vi "SafeMove.vi"(0 "Total Distance (mm)":dbl, 5 "Forward/Reverse":bool, 7 "Calibration Constant":dbl, 9 "Axis#":i16 min=0 max=2 step=1) -> (11 "5V Indicator":bool)   [LabVIEW 2017]
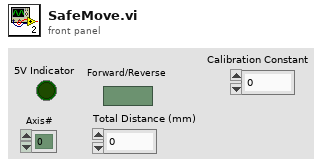
[diagram p1: front panel]
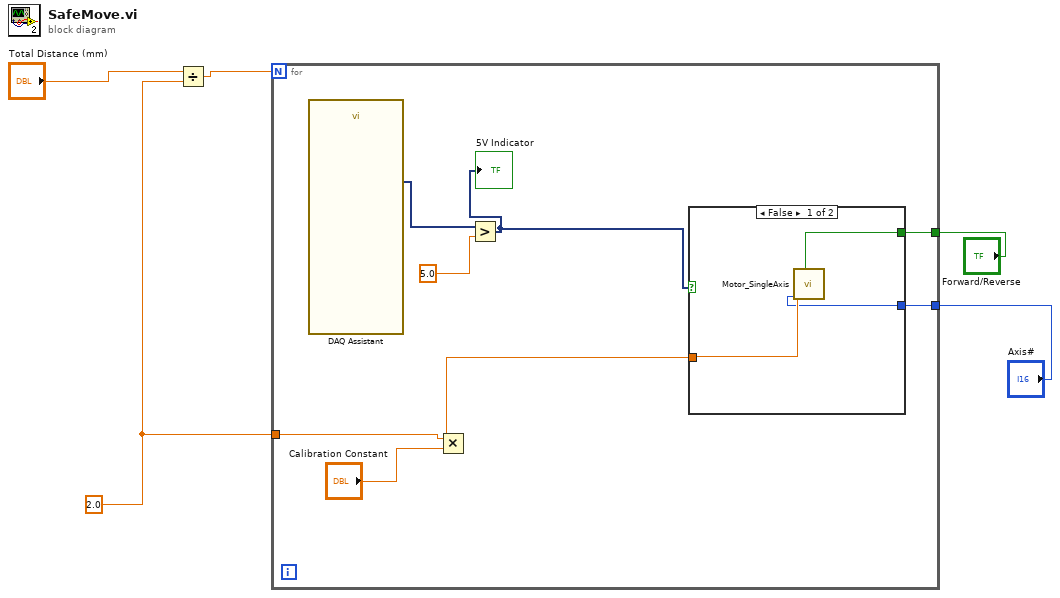
[diagram p0: block diagram]
diagram:
  w3 = 2.0 ("y")
  n1 = Divide(x="Total Distance (mm)", y=w3) -> (x/y=w5:dbl)
  n2 = for {
    N: w5 -> [_]
    tunnel: w3 -> [w10]
    tunnel: "Forward/Reverse" -> [w9]
    tunnel: "Axis#" -> [w8]
    n3 = call "DAQ Assistant"() -> ("data"=w7:dynamicdata)  [unwired: 17 in, 2 out]
    n4 = Multiply(x=w10, y="Calibration Constant") -> (x*y=w12:dbl)
    n5 = Greater?(x=w7, y=5.0) -> (0:w11:dynamicdata)
    "5V Indicator" <- w11
    n6 = case shown="False" w11 {
      tunnel: w12 -> [w16 _]
      tunnel: w9 -> [w15 _]
      tunnel: w8 -> [w14 _]
      frame False {
        n7 = call <userlib>:"Motor_SingleAxis.vi"("# of Steps (x100)"=w16, "Axis#"=w14, "Forward/Reverse"=w15) -> ()  [unwired: 2 in, 2 out]
      }
      frame True {
      }
    }
  }
